vi "PowerElecControl.vi"(8 "error in":errorcluster caption="错误输入", 10 "设置通道开关":bool[](array[boolean])=[FALSE, TRUE, FALSE, TRUE], 11 "线":tag="Dev9/port0/line0:3") -> (0 "error out":errorcluster caption="错误输出")   [LabVIEW 2014, in "HardWareConfig.lvlib"]
doc: "该范例演示了如何连续重新生成数字输出数据。该输出为硬件定时，因此每个采样均在下一个采样时钟滴答输出。\n\n某些硬件（例如，M系列DAQ）必须使用外部采样时钟实现数字任务。如要查看可用的采样时钟源的完整列表，见Measurement and Automation Explorer的设备连线表。\n\n关于连线信号至DAQ设备的操作指南，请查看设备文档。"
uses:
  HardWareConfig.lvlib
  <vilib>/DAQmx/write.llb/DAQmx Write (Digital 1D Bool 1Chan 1Samp).vi
  <vilib>/DAQmx/create/channels.llb/DAQmx Create Channel (DO-Digital Output).vi
  <vilib>/DAQmx/miscellaneous.llb/DAQmx Fill In Error Info.vi
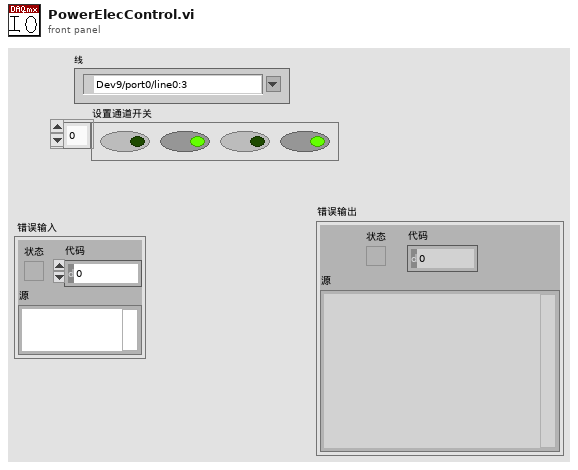
[diagram p1: front panel]
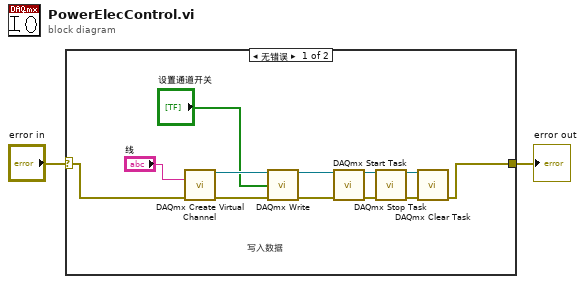
[diagram p0: block diagram]
diagram:
  n1 = case shown="无错误" "error in" {
    selector: "error in" -> [w4 w15]
    tunnel: [w3 w15] -> w1
    frame No Error {
      # "写入数据"
      n2 = call-poly <vilib>:"DAQmx Create Virtual Channel.vi"("lines"="线", "error in"=w4) -> ("task out"=w9:refnum<k21>, "error out"=w8:errorcluster)  [unwired: 12 in]
      n3 = call-poly <vilib>:"DAQmx Write.vi"("task/channels in"=w9, "data"="设置通道开关", "error in"=w8) -> ("task out"=w14:refnum<k21>, "error out"=w13:errorcluster)  [unwired: 10 in, 1 out]
      n4 = call <vilib>:"DAQmx Start Task.vi"("task/channels in"=w14, "error in"=w13) -> ("task out"=w6:refnum<k21>, "error out"=w5:errorcluster)  [unwired: 12 in]
      n5 = call <vilib>:"DAQmx Stop Task.vi"("task/channels in"=w6, "error in"=w5) -> ("task out"=w11:refnum<k21>, "error out"=w10:errorcluster)  [unwired: 12 in]
      n6 = call <vilib>:"DAQmx Clear Task.vi"("task in"=w11, "error in"=w10) -> ("error out"=w3:errorcluster)  [unwired: 13 in]
    }
    frame Error {
    }
  }
  "error out" <- w1
